vi "Open HTML Report in Browser.vi"   [LabVIEW 2017, in "NI_ReportGenerationCore.lvlib"]
doc: "Displays an HTML report in the default Web browser. Wire data to the <B>report in</B> input to determine the polymorphic instance to use or manually select the instance. You cannot use this VI with standard reports."
uses:
  <vilib>/Utility/NIReport.llb/NI_ReportGenerationCore.lvlib
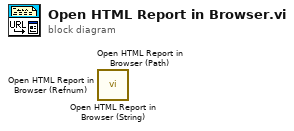
[diagram p0: block diagram]
diagram:
  n1 = call <vilib>:"Open HTML Report in Browser (String).vi"() -> ()  [unwired: 14 in, 2 out]
  n2 = call <vilib>:"Open HTML Report in Browser (Path).vi"() -> ()  [unwired: 14 in, 2 out]
  n3 = call <vilib>:"Open HTML Report in Browser (Refnum).vi"() -> ()  [unwired: 13 in, 3 out]
